vi "startDriveMode.vi"(8 "error in (no error)":errorcluster, 9 "interface object in":refnum<k20>, 11 "MotorControllerClass in":refnum<class "MotorControllerClass.lvclass">) -> (0 "error out":errorcluster, 1 "interface object out":refnum<k20>, 2 "startDriveRes":u32, 3 "MotorControllerClass out":refnum<class "MotorControllerClass.lvclass">)   [LabVIEW 2018, in "MotorControllerClass.lvclass"]
uses:
  BMS/MotorControllerClass.lvclass
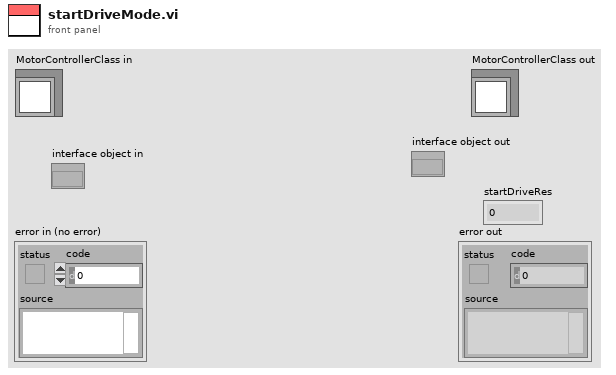
[diagram p1: front panel]
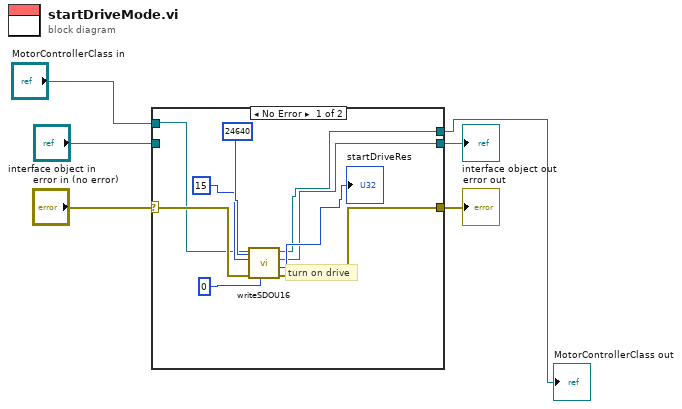
[diagram p0: block diagram]
diagram:
  n1 = case shown="No Error" "error in (no error)" {
    selector: "error in (no error)" -> [w13 w18]
    tunnel: [w12 w18] -> w5
    tunnel: [w9 w16] -> w1
    tunnel: "interface object in" -> [_ w17]
    tunnel: [w10 w17] -> w3
    tunnel: "MotorControllerClass in" -> [w7 w16]
    frame No Error {
      # "turn on drive"
      n2 = call "writeSDOU16.vi"("object sub-index (0)"=u8 0, "object index"=u16 24640, "error in (no error)"=w13, "inputNumber"=u16 15, "MotorControllerClass in"=w7) -> ("error out"=w12:errorcluster, "completion code"=→"startDriveRes":u32, "interface object out"=w10:refnum<k20>, "MotorControllerClass out"=w9:refnum<class "MotorControllerClass.lvclass">)  [unwired: 3 in]
    }
    frame Error {
    }
  }
  "error out" <- w5
  "interface object out" <- w3
  "MotorControllerClass out" <- w1
